vi "Cash Card Map History.vi"() -> ()   [LabVIEW 2021]
uses:
  6fb0b00a-45ef-4051-b8b4-4a683b7d636f.vi
panel:
  in  "stop":bool
  in  "Tab Control":enum32{"Dealt Card Map", "Shown Card Maps"}(tab)
  out "Card Map (Dealt)":T1(array[cluster]) {"Average Profit/Loss (BBs)" format="%#_3g"}
  out "Overall Profit/Loss (BBs)":dbl
  out "Total Hands":i32
  out "Profit per Hand Dealt":dbl=nan format="%#_3g"
  in  "Player":u16(ring) items=["Jonathan-M", "Andrew", "Mark", "Tom", "Ian", "Marty", "Jeff-T", "Dennis", "Jonathan-H", "Ethan", "Brian", "Erik", "Ira", "Gregg"]
  out "Card Map (Shown)":T1(array[cluster]) {"Average Profit/Loss (BBs)" format="%#_3g"}
  out "Overall Profit/Loss (BBs, Shown)":dbl
  out "Total Hands (Shown)":i32
  out "Profit per Hand Shown":dbl=nan format="%#_3g"
  out "Slide":u16(slide) scale=0.0..25.0
  out "Number of Files":i32
  in  "File Filter Pattern":string="*C.txt"
  in  "Path to hand history files":path=path "C:/Users/manma/Google Drive/WPC Stat Scrape/Data/Hand Histories"
  # "SUITED"
  # "OFFSUIT"
  # "A"
  # "K"
  # "Q"
  # "J"
  # "T"
  # "9"
  # "8"
  # "7"
  # "6"
  # "5"
  # "4"
  # "3"
  # "2"
  # "2"
  # "3"
  # "4"
  # "5"
  # "6"
  # "7"
  # "8"
  # "9"
  # "T"
  # "J"
  # "Q"
  # "K"
  # "A"
  # "A"
  # "K"
  # "Q"
  # "J"
  # "T"
  # "9"
  # "8"
  # "7"
  # "6"
  # "5"
  # "4"
  # "3"
  # "2"
  # "2"
  # "3"
  # "4"
  # "5"
  # "6"
  # "7"
  # "8"
  # "9"
  # "T"
  # "J"
  # "Q"
  # "K"
  # "A"
  # "SUITED"
  # "OFFSUIT"
  # "A"
  # "K"
  # "Q"
  # "J"
  # "T"
  # "9"
  # "8"
  # "7"
  # "6"
  # "5"
  # "4"
  # "3"
  # "2"
  # "2"
  # "3"
  # "4"
  # "5"
  # "6"
  # "7"
  # "8"
  # "9"
  # "T"
  # "J"
  # "Q"
  # "K"
  # "A"
  # "A"
  # "K"
  # "Q"
  # "J"
  # "T"
  # "9"
  # "8"
  # "7"
  # "6"
  # "5"
  # "4"
  # "3"
  # "2"
  # "2"
  # "3"
  # "4"
  # "5"
  # "6"
  # "7"
  # "8"
  # "9"
  # "T"
  # "J"
  # "Q"
  # "K"
  # "A"
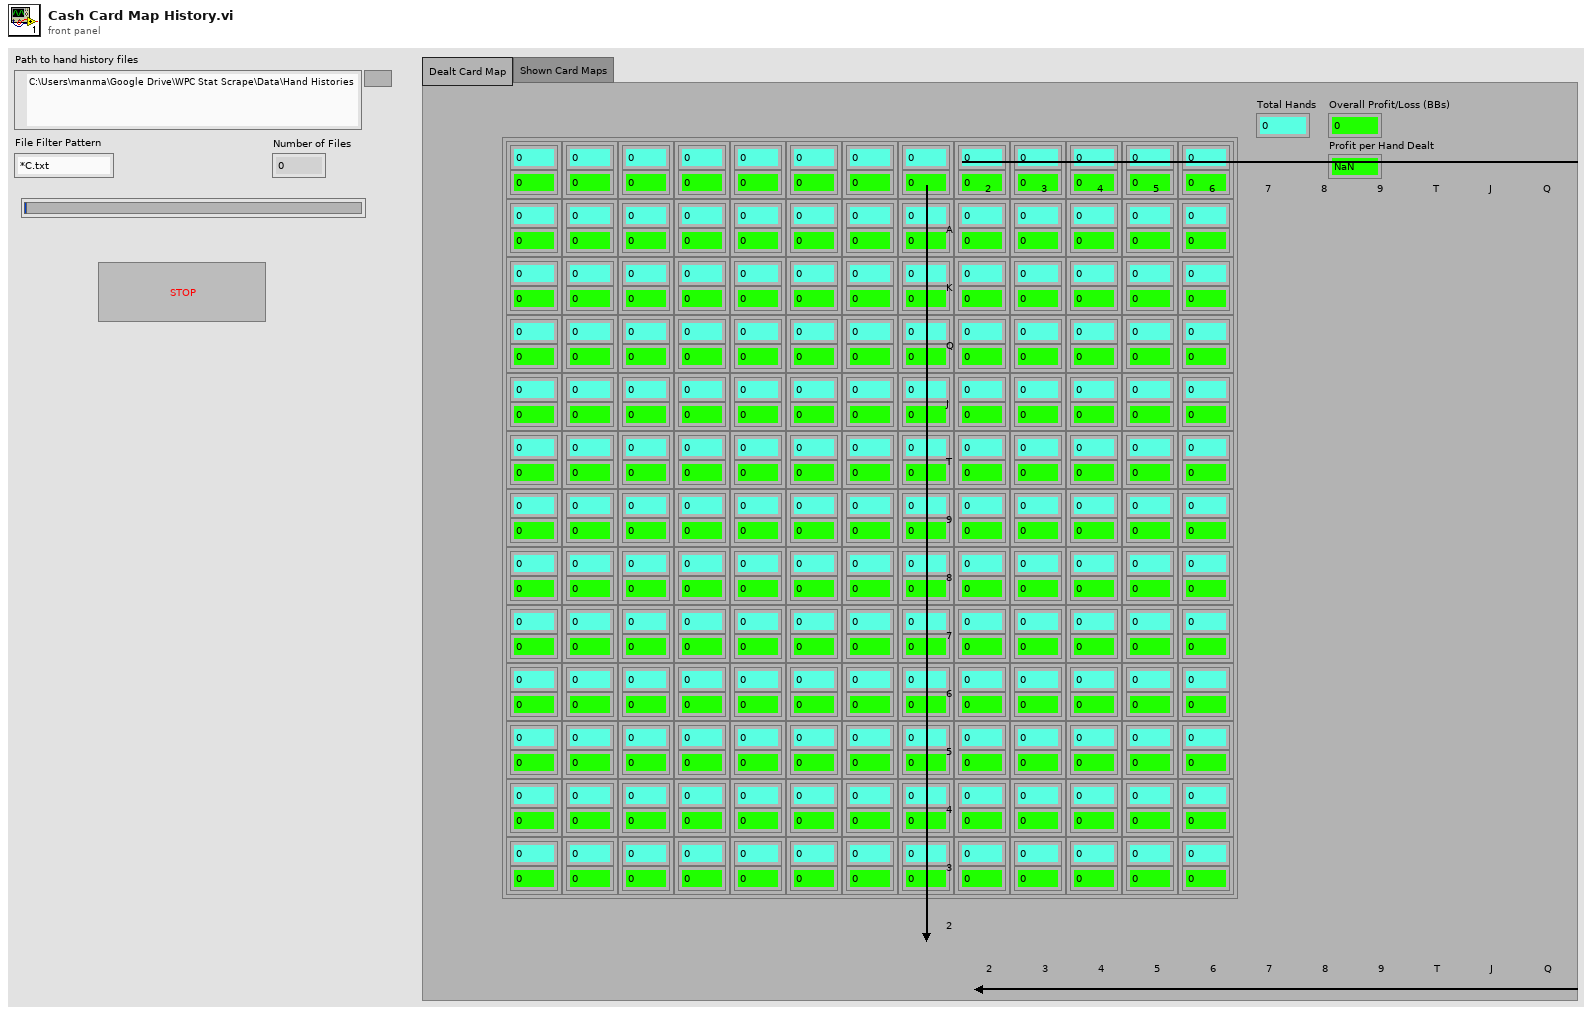
[diagram p1: front panel]
types:
  T1 = cluster{"Hand Count":u16, "Average Profit/Loss (BBs)":dbl}[][]
  T2 = cluster{"Hand Count":u16, "Average Profit/Loss (BBs)":dbl}
  T3 = cluster{"Count":u16, "Profit/Loss (BBs)":dbl}[][]
  T4 = cluster{string, "Card Map":cluster{"Hand Count":u16, "Average Profit/Loss (BBs)":dbl}[][]}
  T5 = cluster{"Hand Count":u16, "Average Profit/Loss (BBs)":dbl}[][][]
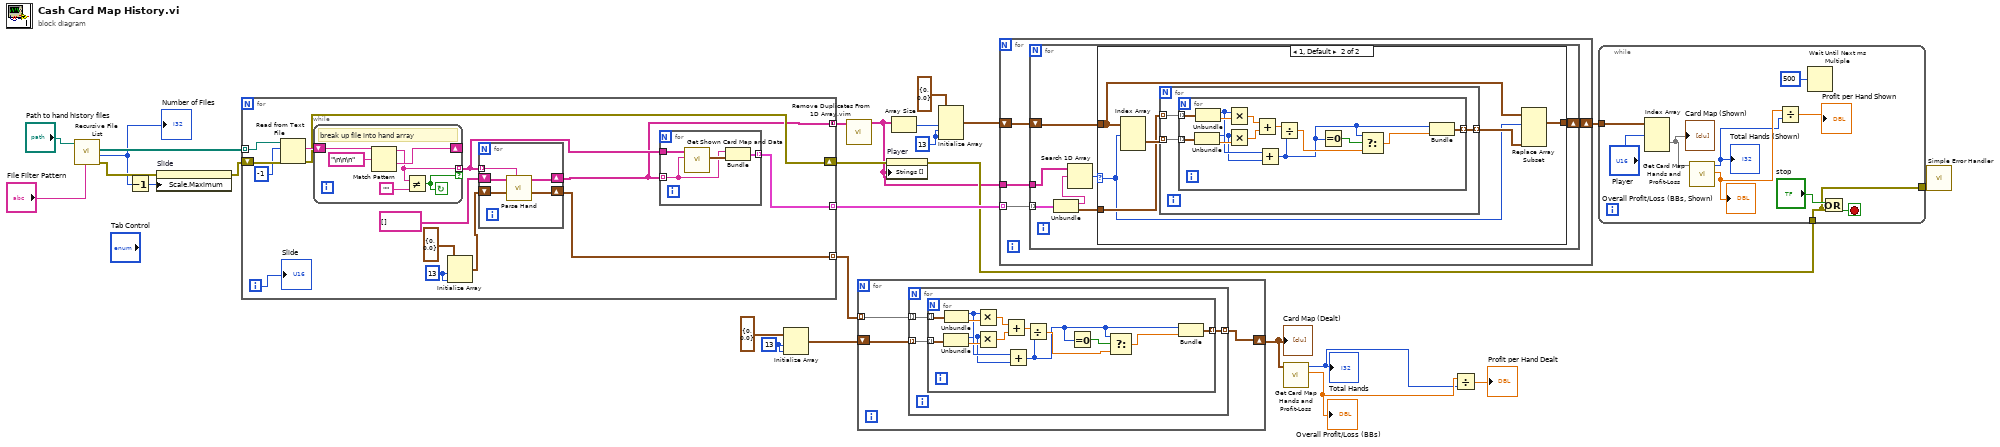
[diagram p0: block diagram]
diagram:
  w11 = 13 ("dimension size")
  w17 = 13 ("dimension size")
  n1 = call <vilib>:"Recursive File List.vi"("pattern"="File Filter Pattern", "Folder Path"="Path to hand history files") -> ("error out"=w23:errorcluster, "Number of Files"=w20:i32, "All Files in Dir"=w24:path[])  [unwired: 5 in, 2 out]
  "Number of Files" <- w20
  n2 = Decrement(x=w20) -> (x-1=w21:i32)
  n3 = property on="Slide" class="Slide (strict)"(error in=w23, "Scale.Maximum"=w21) -> (error out=w22:errorcluster)  [unwired: 1 in, 1 out]
  n4 = for {
    tunnel: w24 -> [w39] mode=indexing
    shift-right: [w31] -> w18
    shift-left: w22 -> [w40]
    tunnel: [w29] -> w19 mode=concatenating
    tunnel: [w28] -> w13 mode=indexing
    tunnel: [w27] -> w10 mode=indexing
    i -> [w30]
    w34 = 13 ("dimension size")
    n5 = Read from Text File(file (use dialog)=w39, count=-1, error in=w40) -> (text=w37:string, error out=w31:errorcluster)  [unwired: 1 in, 2 out]
    n6 = while {
      shift-right: [w54] -> _
      shift-left: w37 -> [w55]
      tunnel: [w52] -> w32 mode=indexing if=w50
      stop <- w50 continue-if-true
      # "break up file into hand array"
      n7 = Match Pattern(string=w55, regular expression="\n\n\n") -> (before substring=w52:string, after substring=w54:string)  [unwired: 1 in, 2 out]
      n8 = Not Equal?(x=w52, y="") -> (x != y?=w50:bool)
    }
    n9 = Initialize Array(T2 {"Hand Count"=0, "Average Profit/Loss (BBs)"=0.0} ("Cluster"), w34, w34) -> (w33:T1)
    n10 = for {
      tunnel: w32 -> [w47] mode=indexing
      shift-right: [w48] -> w29
      shift-left: string[] [] -> [w49]
      shift-right: [w45] -> w28
      shift-left: w33 -> [w46]
      n11 = call "Parse Hand.vi"("Hand History String"=w47, "Card Map In"=w46, "Player Names"=w49) -> ("Card Map Out"=w45:T3, "Player Names Out"=w48:string[])  [unwired: 6 in, 1 out]
    }
    n12 = for {
      tunnel: w32 -> [w44]
      tunnel: w29 -> [w41] mode=indexing
      tunnel: [w43] -> w27 mode=indexing
      n13 = call "Get Shown Card Map and Data.vi"("Player"=w41, "Hand Array"=w44) -> ("Card Map"=w42:T1)  [unwired: 6 in, 3 out]
      n14 = Bundle(w41, "Card Map"=w42) -> (w43:T4)  [unwired: 1 in]
    }
    "Slide" <- w30
  }
  n15 = Initialize Array(T2 {"Hand Count"=0, "Average Profit/Loss (BBs)"=0.0} ("Cluster"), w17, w17) -> (w15:T1)
  n16 = call "Remove Duplicates From 1D Array.vim"("array"=w19) -> ("array with duplicates removed"=w5:string[])  [unwired: 10 in]
  n17 = for {
    shift-right: [w56] -> w14
    shift-left: w15 -> [w57]
    tunnel: w13 -> [w58] mode=indexing
    n18 = for {
      tunnel: w58 -> [w61] mode=indexing
      tunnel: w57 -> [w60] mode=indexing
      tunnel: [w59] -> w56 mode=indexing
      n19 = for {
        tunnel: w61 -> [w75] mode=indexing
        tunnel: w60 -> [w74] mode=indexing
        tunnel: [w73] -> w59 mode=indexing
        n20 = Unbundle(w74) -> ("Hand Count"=w67:u16, "Average Profit/Loss (BBs)"=w72:dbl)
        n21 = Unbundle(w75) -> ("Hand Count"=w68:u16, "Average Profit/Loss (BBs)"=w71:dbl)
        n22 = Multiply(x=w68, y=w71) -> (x*y=w70:dbl)
        n23 = Multiply(x=w67, y=w72) -> (x*y=w69:dbl)
        n24 = Add(x=w70, y=w69) -> (x+y=w66:dbl)
        n25 = Add(x=w68, y=w67) -> (x+y=w63:u16)
        n26 = Divide(x=w66, y=w63) -> (x/y=w64:dbl)
        n27 = Equal To 0?(x=w63) -> (x = 0?=w65:bool)
        n28 = Select(t=w63, s=w65, f=w64) -> (s? t:f=w62:dbl)
        n29 = Bundle(w63, w62) -> (w73:cluster{u16, dbl})  [unwired: 1 in]
      }
    }
  }
  "Card Map (Dealt)" <- w14
  n30 = property on="Player" class="Ring (strict)"(error in=w18, "Strings []"=w5) -> (error out=w8:errorcluster)  [unwired: 1 in, 1 out]
  n31 = Array Size(array=w5) -> (size(s)=w4:i32)
  n32 = Initialize Array(T2 {"Hand Count"=0, "Average Profit/Loss (BBs)"=0.0} ("Cluster"), w4, w11, w11) -> (w9:T5)
  n33 = for {
    tunnel: w10 -> [w79] mode=indexing
    shift-right: [w76] -> w6
    shift-left: w9 -> [w78]
    tunnel: w5 -> [w77]
    n34 = for {
      tunnel: w79 -> [w86] mode=indexing
      tunnel: w77 -> [w82]
      shift-right: [w83] -> w76
      shift-left: w78 -> [w84]
      n35 = Unbundle(w86) -> (w81:string, "Card Map"=w85:T1)
      n36 = Search 1D Array(1D array=w82, element=w81) -> (index of element=w80:i32)  [unwired: 1 in]
      n37 = case shown="1, Default" w80 {
        selector: w80 -> [_ w88]
        tunnel: w85 -> [_ w92]
        tunnel: w84 -> [w87 w91]
        tunnel: [w87 w89] -> w83
        frame -1 {
        }
        frame 1, Default {
          n38 = Index Array(array=w91, index (dim 0)=w88) -> (element=w93:T1)  [unwired: 2 in]
          n39 = for {
            tunnel: w92 -> [w96] mode=indexing
            tunnel: w93 -> [w95] mode=indexing
            tunnel: [w94] -> w90 mode=indexing
            n40 = for {
              tunnel: w96 -> [w110] mode=indexing
              tunnel: w95 -> [w109] mode=indexing
              tunnel: [w108] -> w94 mode=indexing
              n41 = Unbundle(w109) -> ("Hand Count"=w102:u16, "Average Profit/Loss (BBs)"=w107:dbl)
              n42 = Unbundle(w110) -> ("Hand Count"=w103:u16, "Average Profit/Loss (BBs)"=w106:dbl)
              n43 = Multiply(x=w103, y=w106) -> (x*y=w105:dbl)
              n44 = Multiply(x=w102, y=w107) -> (x*y=w104:dbl)
              n45 = Add(x=w105, y=w104) -> (x+y=w101:dbl)
              n46 = Add(x=w103, y=w102) -> (x+y=w98:u16)
              n47 = Divide(x=w101, y=w98) -> (x/y=w99:dbl)
              n48 = Equal To 0?(x=w98) -> (x = 0?=w100:bool)
              n49 = Select(t=w98, s=w100, f=w99) -> (s? t:f=w97:dbl)
              n50 = Bundle(w98, w97) -> (w108:cluster{u16, dbl})  [unwired: 1 in]
            }
          }
          n51 = Replace Array Subset(array=w91, new element=w90, index (dim 0)=w88) -> (w89:T5)  [unwired: 2 in]
        }
      }
    }
  }
  n52 = call "Get Card Map Hands and Profit-Loss.vi"("Card Map In"=w14) -> ("Profit/Loss (BBs)"=w3:dbl, "Total Hands"=w2:i32)  [unwired: 9 in]
  "Total Hands" <- w2
  "Overall Profit/Loss (BBs)" <- w3
  n53 = Divide(x=w3, y=w2) -> (x/y=→"Profit per Hand Dealt":dbl)
  n54 = while {
    tunnel: w6 -> [w120]
    tunnel: w8 -> [w115]
    tunnel: [w115] -> w7
    stop <- w116 stop-if-true
    n55 = Index Array(array=w120, index (dim 0)="Player") -> (element=w118:T1)  [unwired: 2 in]
    "Card Map (Shown)" <- w118
    n56 = call "Get Card Map Hands and Profit-Loss.vi"("Card Map In"=w118) -> ("Profit/Loss (BBs)"=w113:dbl, "Total Hands"=w112:i32)  [unwired: 9 in]
    "Total Hands (Shown)" <- w112
    "Overall Profit/Loss (BBs, Shown)" <- w113
    n57 = Divide(x=w113, y=w112) -> (x/y=→"Profit per Hand Shown":dbl)
    n58 = Wait Until Next ms Multiple(millisecond multiple=u32 500) -> ()  [unwired: 1 out]
    n59 = Or(x="stop", y=w115) -> (x .or. y?=w116:bool)
  }
  n60 = call <vilib>:"Simple Error Handler.vi"("error in (no error)"=w7) -> ()  [unwired: 4 in, 5 out]
